vi "TPNT_StartAsyncServer.vi"(4 "notifier":refnum<notifier>, 5 "updaterate":refnum<vi>, 6 "stop":refnum<vi>, 7 "async":refnum<vi>, 8 "error in (no error)":errorcluster, 10 "port":u16=7000) -> (0 "error out":errorcluster)   [LabVIEW 2016]
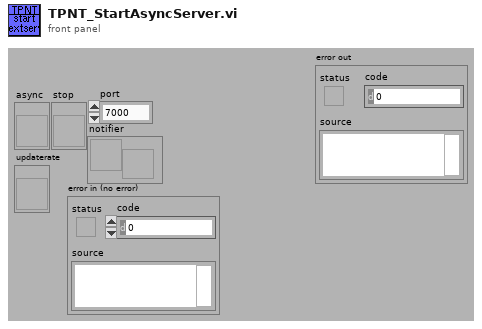
[diagram p1: front panel]
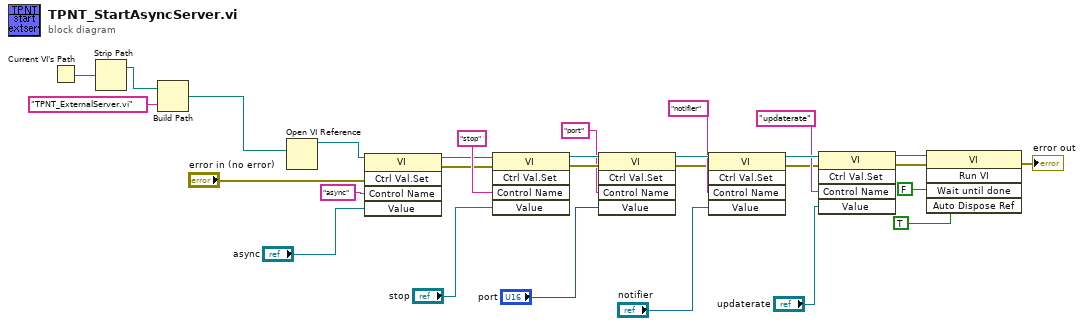
[diagram p0: block diagram]
diagram:
  n1 = Current VI's Path() -> (path=w10:path)
  n2 = Strip Path(path=w10) -> (stripped path=w9:path)  [unwired: 1 out]
  n3 = Build Path(base path=w9, name or relative path="TPNT_ExternalServer.vi") -> (appended path=w7:path)
  n4 = Open VI Reference(vi path=w7) -> (vi reference=w29:refnum<vi>)  [unwired: 1 in, 5 out]
  n5 = invoke class="VI" method="Ctrl Val.Set"(reference=w29, error in="error in (no error)", "Control Name"="async", "Value"="async") -> (reference out=w26:refnum<vi>, error out=w4:errorcluster)  [unwired: 1 in, 3 out]
  n6 = invoke class="VI" method="Ctrl Val.Set"(reference=w26, error in=w4, "Control Name"="stop", "Value"="stop") -> (reference out=w25:refnum<vi>, error out=w24:errorcluster)  [unwired: 1 in, 3 out]
  n7 = invoke class="VI" method="Ctrl Val.Set"(reference=w25, error in=w24, "Control Name"="port", "Value"="port") -> (reference out=w22:refnum<vi>, error out=w3:errorcluster)  [unwired: 1 in, 3 out]
  n8 = invoke class="VI" method="Ctrl Val.Set"(reference=w22, error in=w3, "Control Name"="notifier", "Value"="notifier") -> (reference out=w19:refnum<vi>, error out=w2:errorcluster)  [unwired: 1 in, 3 out]
  n9 = invoke class="VI" method="Ctrl Val.Set"(reference=w19, error in=w2, "Control Name"="updaterate", "Value"="updaterate") -> (reference out=w13:refnum<vi>, error out=w1:errorcluster)  [unwired: 1 in, 3 out]
  n10 = invoke class="VI" method="Run VI"(reference=w13, error in=w1, "Wait until done"=FALSE ("Wait Until Done"), "Auto Dispose Ref"=TRUE ("Auto Dispose Reference")) -> (error out=→"error out":errorcluster)  [unwired: 1 in, 4 out]
